vi "VMUIselfTerminateTest(clientSubpanel).vi"(11 "VariableManagerRef in":refnum<vi>) -> ()   [LabVIEW 2013]
uses:
  VariableManagerCodes/VariableManager/VariableManager.lvclass
  VariableManagerCodes/API/VariableManagerAPI.lvlib
panel:
  in  "Stop":bool
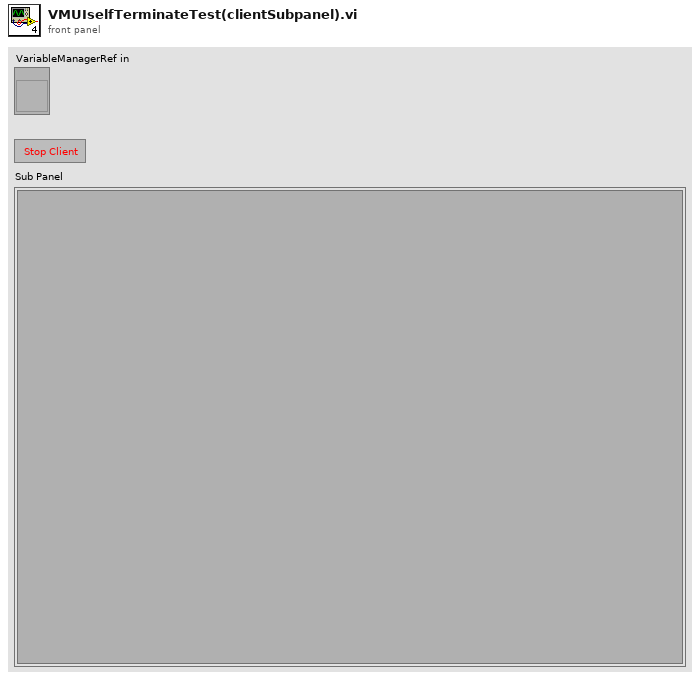
[diagram p1: front panel]
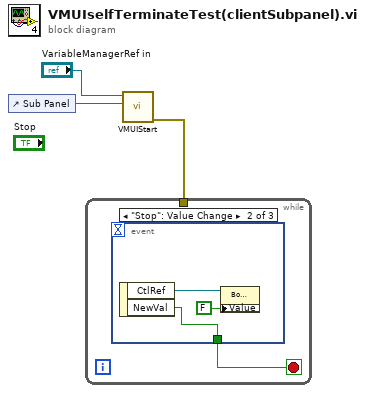
[diagram p0: block diagram]
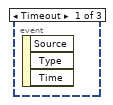
[diagram p2: hidden frame]
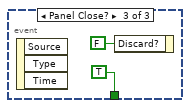
[diagram p3: hidden frame]
diagram:
  n1 = control-ref of="Sub Panel"() -> (w3:refnum<vi>)
  n2 = call "VMUIStart.vi"("SubPanelRef"=w3, "VariableManagerRef in"="VariableManagerRef in") -> ("error out"=w1:errorcluster)  [unwired: 8 in, 1 out]
  n3 = while {
    tunnel: w1 -> [_]
    stop <- w4 stop-if-true
    n4 = event shown="[1] \"Stop\": Value Change" {
      selector: _ -> [_ _ _]
      dyn-events: _ -> [_ _ _]
      timeout: _ -> [_ _ _]
      tunnel: [_ w7 TRUE] -> w4
      event Timeout {
        n5 = event-data() -> ()  [unwired: 1 in, 3 out]
      }
      event "Stop": Value Change {
        n6 = event-data() -> ("CtlRef"=w6:refnum<vi>, "NewVal"=w7:bool)  [unwired: 1 in]
        n7 = property class="Bool (strict)"(reference=w6, "Value"=FALSE) -> ()  [unwired: 1 in, 2 out]
      }
      event Panel Close? {
        n8 = event-data() -> ()  [unwired: 1 in, 3 out]
        n9 = event-data("Discard?"=FALSE) -> ()  [unwired: 1 in, 1 out]
      }
    }
  }
